vi "SVPO Order Metrics for Periodic Inspection (N Ch).vi"(0 "even-angle signals":cluster{"r0":dbl, "dr":dbl, "Y":dbl[]}[](array[cluster]) {"r0" format="%.2p"; "dr" format="%.2p"; "Y" format="%.2f"}, 1 "update? (T)":bool=TRUE, 2 "reset? (F)":bool, 7 "even-angle position info":T2, 9 "orders":dbl[](array[numeric])=[1.0] format="%.2f", 11 "integration cycles":u32=8, 12 "measurement selection":T1={"speed"=TRUE, "DC gap"=TRUE, "RMS level"=TRUE, "max-min level"=TRUE, "magnitude"=TRUE, "phase"=TRUE}) -> (3 "speed [RPM]":dbl, 4 "DC gap":dbl[](array[numeric]), 6 "RMS level":dbl[](array[numeric]), 8 "max-min level":dbl[](array[numeric]), 10 "magnitudes [RMS]":dbl[][](array[numeric]), 15 "phase [phase lag]":dbl[][](array[numeric]))   [LabVIEW 2017, in "SoundVib_OrderTracking.lvlib"]
doc: "Computes the metrics of designated orders in an even-angle signal, such as magnitudes, phases, speed, DC gap, RMS level, and max-min level. This VI calculates metrics values from the latest integration cycles of the even-angle signal. Use this VI on embedded targets that have limited computational resources. Wire data to the <B>even-angle signal</B> input to determine the polymorphic instance to use or manually select the instance."
uses:
  <vilib>/addons/Sound and Vibration/Order Analysis/Resample Order Tracking/SoundVib_OrderTracking.lvlib
  <vilib>/addons/Sound and Vibration/Order Analysis/Misc/OAT Position Info.ctl
  <vilib>/Analysis/baseanly.llb/Mean (DBL).vi
  <vilib>/Analysis/5stat.llb/RMS (DBL).vi
  <vilib>/addons/Sound and Vibration/Order Analysis/Resample Order Tracking/SubVIs/sv_Buffer Even-Angle Signal (1 Ch).vi
  <vilib>/Analysis/NI_AALPro.lvlib
  <vilib>/Analysis/NI_AALBase.lvlib
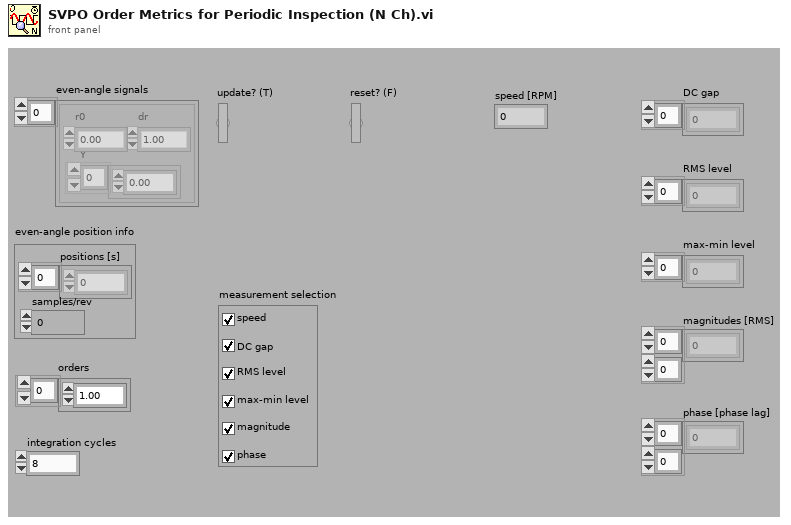
[diagram p1: front panel]
types:
  T1 = cluster{"speed":bool, "DC gap":bool, "RMS level":bool, "max-min level":bool, "magnitude":bool, "phase":bool}
  T2 = typedef "OAT Position Info.ctl" = cluster{"positions [s]":dbl[], "samples/rev":dbl}
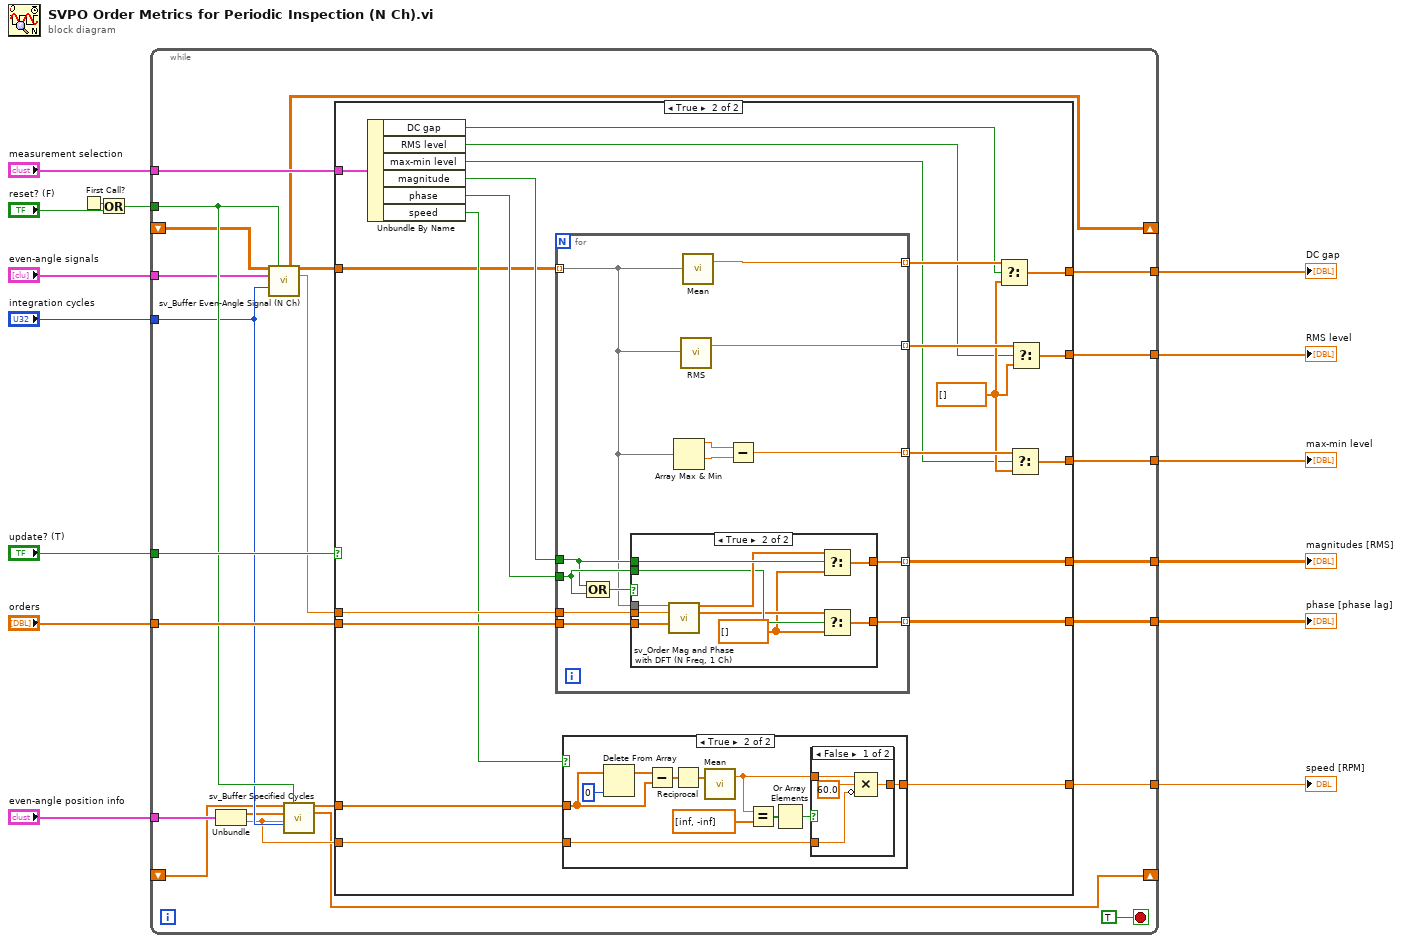
[diagram p0: block diagram]
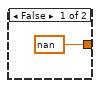
[diagram p2: hidden frame]
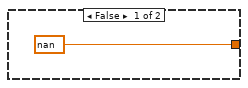
[diagram p4: hidden frame]
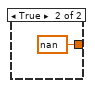
[diagram p5: hidden frame]
diagram:
  n1 = First Call?() -> (First Call?: T/F=w14:bool)
  n2 = Or(x=w14, y="reset? (F)") -> (x .or. y?=w3:bool)
  n3 = while {
    tunnel: "orders" -> [w38]
    tunnel: [w36] -> w12
    tunnel: [w35] -> w11
    tunnel: "update? (T)" -> [w34]
    tunnel: "even-angle signals" -> [w19]
    tunnel: [w32] -> w8
    tunnel: [w31] -> w7
    tunnel: [w30] -> w6
    tunnel: "measurement selection" -> [w29]
    tunnel: "even-angle position info" -> [w28]
    tunnel: w3 -> [w27]
    tunnel: "integration cycles" -> [w26]
    tunnel: [w24] -> w1
    shift-right: [w16] -> _
    shift-left: _ -> [w21]
    shift-right: [w17] -> _
    shift-left: _ -> [w18]
    stop <- TRUE stop-if-true
    n4 = Unbundle(w28) -> ("positions [s]"=w22:dbl[], "samples/rev"=w20:dbl)
    n5 = call <vilib>:"sv_Buffer Even-Angle Signal (N Ch).vi"("initial buffered x[n]"=w18, "reset? (True)"=w27, "even-angle signals"=w19, "integration cycles"=w26) -> ("buffered x[n]"=w17:dbl[][], "buffered x[n] for analysis"=w37:dbl[][], "sample rate"=w33:dbl)  [unwired: 9 in]
    n6 = call <vilib>:"sv_Buffer Specified Cycles.vi"("inital buffered x[n]"=w21, "reset? (True)"=w27, "x[n]"=w22, "fs"=w20, "integration cycles"=w26) -> ("buffered x[n] for analysis"=w25:dbl[], "buffered x[n]"=w16:dbl[])  [unwired: 9 in]
    n7 = case shown="True" w34 {
      tunnel: w29 -> [_ w61]
      tunnel: [_ w50] -> w32
      tunnel: [_ w46] -> w31
      tunnel: w38 -> [_ w60]
      tunnel: w33 -> [_ w59]
      tunnel: w37 -> [_ w40]
      tunnel: [_ w57] -> w36
      tunnel: [_ w56] -> w35
      tunnel: w25 -> [_ w41]
      tunnel: [nan ("mean") w54] -> w24
      tunnel: [_ w45] -> w30
      tunnel: w20 -> [_ w52]
      frame False {
      }
      frame True {
        w44 = dbl[] [] ("f")
        n8 = Unbundle By Name(w61) -> ("DC gap"=w49:bool, "RMS level"=w43:bool, "max-min level"=w42:bool, "magnitude"=w53:bool, "phase"=w58:bool, "speed"=w55:bool)
        n9 = for {
          tunnel: [w74] -> w51 mode=indexing
          tunnel: [w73] -> w47 mode=indexing
          tunnel: w60 -> [w71]
          tunnel: w59 -> [w70]
          tunnel: w58 -> [w69]
          tunnel: [w68] -> w57 mode=indexing
          tunnel: [w67] -> w56 mode=indexing
          tunnel: w53 -> [w66]
          tunnel: w40 -> [w65] mode=indexing
          tunnel: [w64] -> w48 mode=indexing
          n10 = Compound Arithmetic op=OR(w66, w69) -> (w72:bool)
          n11 = case shown="True" w72 {
            tunnel: w71 -> [_ w84]
            tunnel: w70 -> [_ w83]
            tunnel: w65 -> [_ w82]
            tunnel: w66 -> [_ w81]
            tunnel: w69 -> [_ w79]
            tunnel: [_ w76] -> w68
            tunnel: [_ w75] -> w67
            frame False {
            }
            frame True {
              w77 = dbl[] [] ("f")
              n12 = call <vilib>:"sv_Order Mag and Phase with DFT (N Freq, 1 Ch).vi"("buffered x[n]"=w82, "fs"=w83, "fc [Hz]"=w84) -> ("mag [RMS]"=w80:dbl[], "phase"=w78:dbl[])  [unwired: 11 in]
              n13 = Select(t=w80, s=w81, f=w77) -> (s? t:f=w76:dbl[])
              n14 = Select(t=w78, s=w79, f=w77) -> (s? t:f=w75:dbl[])
            }
          }
          n15 = Array Max & Min(array=w65) -> (max value=w63:dbl, min value=w62:dbl)  [unwired: 2 out]
          n16 = call-poly <vilib>:"RMS.vi"("X"=w65) -> ("rms value"=w73:dbl)  [unwired: 1 out]
          n17 = call-poly <vilib>:"Mean.vi"("X"=w65) -> ("mean"=w74:dbl)  [unwired: 1 out]
          n18 = Subtract(x=w63, y=w62) -> (x-y=w64:dbl)
        }
        n19 = case shown="True" w55 {
          tunnel: w41 -> [_ w93]
          tunnel: [nan w94] -> w54
          tunnel: w52 -> [_ w90]
          frame False {
          }
          frame True {
            n20 = Delete From Array(array=w93, index=0) -> (array with subset deleted=w95:dbl[])  [unwired: 1 in, 1 out]
            n21 = Subtract(x=w95, y=w93) -> (x-y=w92:dbl[])
            n22 = Reciprocal(x=w92) -> (1/x=w91:dbl[])
            n23 = call-poly <vilib>:"Mean.vi"("X"=w91) -> ("mean"=w89:dbl)  [unwired: 1 out]
            n24 = Equal?(x=w89, y=dbl[] [inf, -inf]) -> (x = y?=w87:bool[])
            n25 = Or Array Elements(Boolean array=w87) -> (logical OR=w86:bool)
            n26 = case shown="False" w86 {
              tunnel: w89 -> [w100 _]
              tunnel: [w98 nan] -> w94
              tunnel: w90 -> [w97 _]
              frame False {
                n27 = Compound Arithmetic op=MULTIPLY(w100, 60.0 ("y"), invert w97) -> (w98:dbl)
              }
              frame True {
              }
            }
          }
        }
        n28 = Select(t=w51, s=w49, f=w44) -> (s? t:f=w50:dbl[])
        n29 = Select(t=w48, s=w42, f=w44) -> (s? t:f=w45:dbl[])
        n30 = Select(t=w47, s=w43, f=w44) -> (s? t:f=w46:dbl[])
      }
    }
  }
  "magnitudes [RMS]" <- w12
  "phase [phase lag]" <- w11
  "speed [RPM]" <- w1
  "DC gap" <- w8
  "RMS level" <- w7
  "max-min level" <- w6
